vi "Cleanup Path Group.vi"(0 "Path Group in":refnum<class "Path Group.lvclass">, 5 "Path Callback References":refnum<vi>[](array[refnum]), 11 "error in":errorcluster) -> (4 "Path Group out":refnum<class "Path Group.lvclass">, 15 "error out":errorcluster)   [LabVIEW 2023, in "RFFixtureCharact.Public.lvlib"]
uses:
  RFFixtureCharact.Public.lvlib
  Common/Base Classes/Path Group/Path Group.lvclass
  Common/Base Classes/Path/Path.lvclass
  Common/RFCalAndFixtureCharact.Common.lvlib
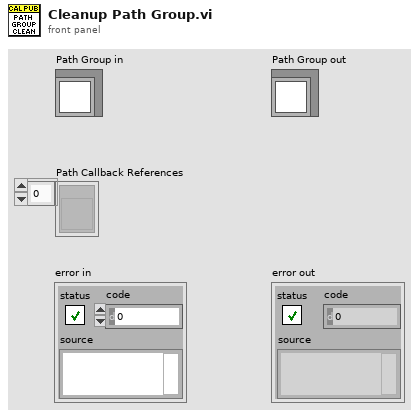
[diagram p1: front panel]
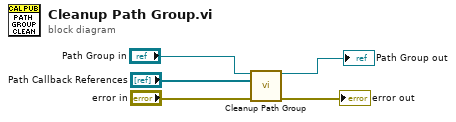
[diagram p0: block diagram]
diagram:
  n1 = call "Cleanup Path Group.vi"("Path Group in"="Path Group in", "Path Callbacks Reference"="Path Callback References", "error in"="error in") -> ("Path Group out"=→"Path Group out":refnum<class "Path Group.lvclass">, "error out"=→"error out":errorcluster)  [unwired: 11 in]
